vi "DSF.Engine.Interface.Get Debug Flags.vi"(11 "Interface in":refnum<class "DSF.Engine.Interface.lvclass">) -> (2 "FIFO Debug Flags":refnum<class "DSF.Engine.Debug Flags.FIFO.lvclass">, 3 "Interface out":refnum<class "DSF.Engine.Interface.lvclass">)   [LabVIEW 2017, in "DSF.Engine.lvlib" / "DSF.Engine.Interface.lvclass"]
uses:
  DSF.Engine.Interface.lvclass
  Debug/DSF.Engine.Debug Flags.FIFO.lvclass
  DSF.Engine.Interface.lvclass/DSF.Engine.Interface.ctl
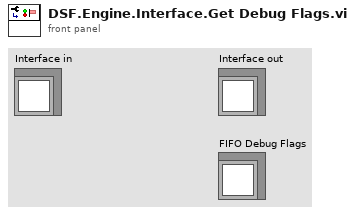
[diagram p1: front panel]
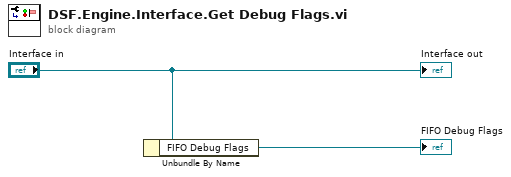
[diagram p0: block diagram]
diagram:
  n1 = Unbundle By Name("Interface in") -> ("FIFO Debug Flags"=→"FIFO Debug Flags":refnum<class "DSF.Engine.Debug Flags.FIFO.lvclass">)
  "Interface out" <- "Interface in"
